vi "filter table.vi"(7 "display column?":bool[](array[boolean]), 8 "error in (no error)":errorcluster, 10 "Sort Types":string[](array[string]), 11 "resource table in":string[][](array[string])) -> (0 "error out":errorcluster, 1 "max string length in columns":i32[](array[numeric]), 2 "Headers":string[](array[string]), 3 "resource table out":string[][](array[string]))   [LabVIEW 2016, in "FPGA Resource Manager System Definition.lvlib"]
uses:
  FPGA Resource Manager System Definition.lvlib
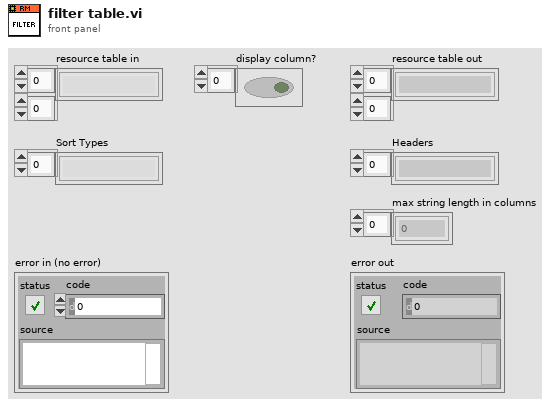
[diagram p1: front panel]
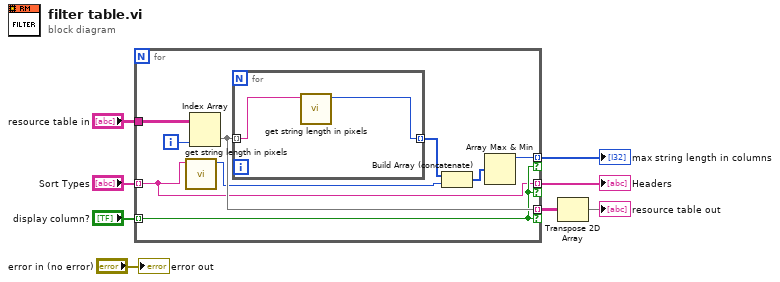
[diagram p0: block diagram]
diagram:
  n1 = for {
    tunnel: "display column?" -> [w11] mode=indexing
    tunnel: "Sort Types" -> [w10] mode=indexing
    tunnel: [w10] -> w6 mode=indexing if=w11
    tunnel: [w15] -> w7 mode=indexing if=w11
    tunnel: "resource table in" -> [w17]
    tunnel: [w14] -> w1 mode=indexing if=w11
    i -> [w16]
    n2 = call "get string length in pixels.vi"("notes"=w10) -> ("Numeric"=w9:i16)  [unwired: 10 in]
    n3 = Index Array(array=w17, index (col)=w16) -> (element=w15:string[])  [unwired: 1 in]
    n4 = for {
      tunnel: w15 -> [w19] mode=indexing
      tunnel: [w18] -> w13 mode=indexing
      n5 = call "get string length in pixels.vi"("notes"=w19) -> ("Numeric"=w18:i16)  [unwired: 10 in]
    }
    n6 = Build Array (concatenate)(w13, w9) -> (w12:i16[])
    n7 = Array Max & Min(array=w12) -> (max value=w14:i16)  [unwired: 3 out]
  }
  "Headers" <- w6
  "max string length in columns" <- w1
  n8 = Transpose 2D Array(2D array=w7) -> (transposed array=→"resource table out":string[][])
  "error out" <- "error in (no error)"
